vi "KMCS2000 DataStringToArray.vi"(11 "read buffer":string) -> (3 "Array":dbl[](array[numeric]))   [LabVIEW 2018]
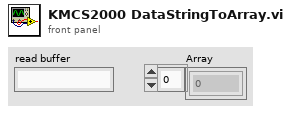
[diagram p1: front panel]
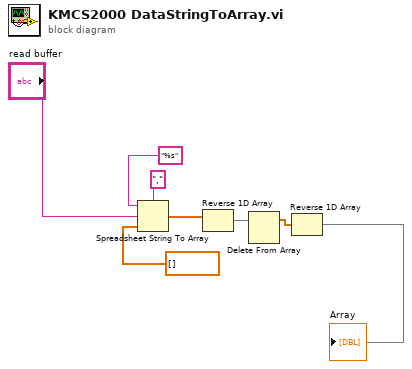
[diagram p0: block diagram]
diagram:
  n1 = Spreadsheet String To Array(delimiter (Tab)=",", format string="%s", spreadsheet string="read buffer", array type (2D Dbl)=dbl[] []) -> (array=w5:dbl[])
  n2 = Reverse 1D Array(array=w5) -> (reversed array=w6:dbl[])
  n3 = Delete From Array(array=w6) -> (array with subset deleted=w7:dbl[])  [unwired: 2 in, 1 out]
  n4 = Reverse 1D Array(array=w7) -> (reversed array=→"Array":dbl[])
